vi "Animation Background Thread.vi"(8 "error in (no error)":errorcluster) -> (0 "error out":errorcluster)   [LabVIEW 2017, in "3D Comet.lvclass"]
uses:
  <vilib>/Math Plots/3D Math Plots/3D Comet/3D Comet/3D Comet.lvclass
  <vilib>/Utility/miscctls.llb/LV3DPointTypeDef.ctl
panel:
  in  "Color Array":cluster{"R":sgl, "G":sgl, "B":sgl, "A":sgl}[](array[cluster])
  in  "Body Object":refnum<vi>
  in  "Vertex Array":cluster{"X":sgl, "Y":sgl, "Z":sgl}[](array[cluster])
  in  "3D Scene Ref":refnum<vi>
  in  "Head Object":refnum<vi>
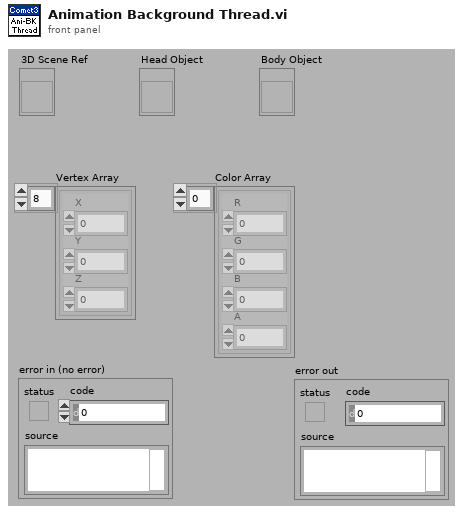
[diagram p1: front panel]
types:
  T1 = typedef "LV3DPointTypeDef.ctl" = cluster{"X":sgl, "Y":sgl, "Z":sgl}
  T2 = enum16{"Overall", "Per Primitive", "Per Vertex", "Binding Off"}
  T3 = enum16{"Points", "Lines", "Line Strip", "Line Loop", "Triangles", "Triangle Strip", "Triangle Fan", "Quads", "Quad Strip", "Polygon"}
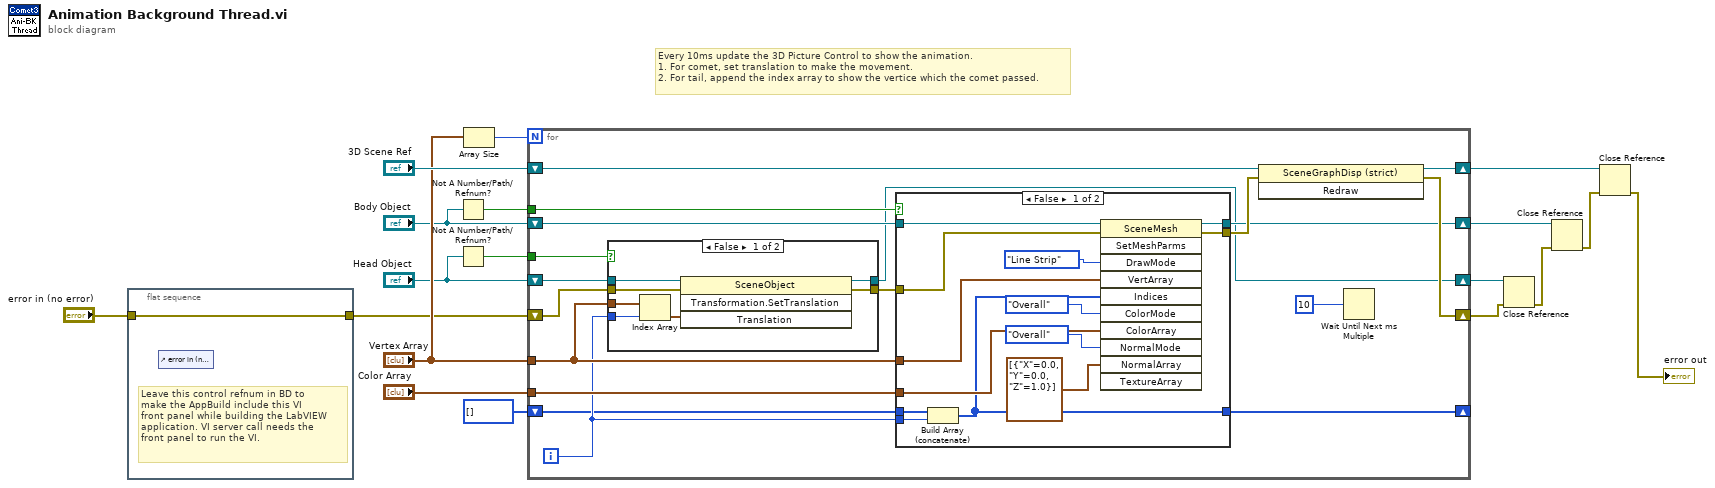
[diagram p0: block diagram]
diagram:
  # "Every 10ms update the 3D Picture Control to show the animation.\n1. For comet, set translation to make the movement.\n2. For tail, append the index array to show the vertice which the comet passed."
  n1 = flat-sequence {
    tunnel: [w19] -> w2
    tunnel: "error in (no error)" -> [w19]
    frame #0 {
      # "Leave this control refnum in BD to \nmake the AppBuild include this VI\nfront panel while building the LabVIEW\napplication. VI server call needs the \nfront panel to run the VI."
      n2 = control-ref of="error in (no error)"() -> ()  [unwired: 1 out]
    }
  }
  n3 = Not A Number/Path/Refnum?(number/path/refnum="Body Object") -> (NaN/Path/Refnum?=w10:bool)
  n4 = Not A Number/Path/Refnum?(number/path/refnum="Head Object") -> (NaN/Path/Refnum?=w11:bool)
  n5 = Array Size(array="Vertex Array") -> (size(s)=w15:i32)
  n6 = for {
    N: w15 -> [_]
    tunnel: "Vertex Array" -> [w33]
    tunnel: "Color Array" -> [w32]
    shift-right: [w25] -> w6
    shift-left: w2 -> [w31]
    shift-right: [w28] -> _
    shift-left: i32[] [] -> [w29]
    tunnel: w11 -> [w24]
    tunnel: w10 -> [w23]
    shift-right: [w22] -> w8
    shift-left: "Body Object" -> [w34]
    shift-right: [w21] -> w9
    shift-left: "3D Scene Ref" -> [w27]
    shift-right: [w20] -> w7
    shift-left: "Head Object" -> [w37]
    i -> [w30]
    n7 = case shown="False" w24 {
      tunnel: w37 -> [w60 w61]
      tunnel: [w59 w62] -> w35
      tunnel: w33 -> [w58 _]
      tunnel: w31 -> [w57 w62]
      tunnel: w30 -> [w55 _]
      tunnel: [w54 w61] -> w20
      frame False {
        n8 = Index Array(array=w58, index=w55) -> (element=w56:cluster{"X":sgl, "Y":sgl, "Z":sgl})
        n9 = invoke class="SceneObject" method="Transformation.SetTranslation"(reference=w60, error in=w57, "Translation"=w56) -> (reference out=w54:refnum<vi>, error out=w59:errorcluster)  [unwired: 1 in, 2 out]
      }
      frame True {
      }
    }
    n10 = case shown="False" w23 {
      tunnel: w35 -> [w50 w52]
      tunnel: w34 -> [w49 w51]
      tunnel: w33 -> [w47 _]
      tunnel: w32 -> [w46 _]
      tunnel: w30 -> [w44 _]
      tunnel: w29 -> [w43 w53]
      tunnel: [w42 w53] -> w28
      tunnel: [w41 w52] -> w26
      tunnel: [w38 w51] -> w22
      frame False {
        n11 = Build Array (concatenate)(w43, w44) -> (w42:i32[])
        n12 = invoke class="SceneMesh" method="SetMeshParms"(reference=w49, error in=w50, "DrawMode"=T3."Line Strip" ("Draw Mode"), "VertArray"=w47, "Indices"=w42, "ColorMode"=T2."Overall" ("Color Binding Mode"), "ColorArray"=w46, "NormalMode"=T2."Overall" ("Normal Binding Mode"), "NormalArray"=T1[] [{"X"=0.0, "Y"=0.0, "Z"=1.0}] ("Normal Array")) -> (reference out=w38:refnum<vi>, error out=w41:errorcluster)  [unwired: 2 in, 9 out]
      }
      frame True {
      }
    }
    n13 = invoke class="SceneGraphDisp (strict)" method="Redraw"(reference=w27, error in=w26) -> (reference out=w21:refnum<vi>, error out=w25:errorcluster)  [unwired: 1 in, 1 out]
    n14 = Wait Until Next ms Multiple(millisecond multiple=u32 10 ("milliseconds to wait")) -> ()  [unwired: 1 out]
  }
  n15 = Close Reference(reference=w7, error in (no error)=w6) -> (error out=w5:errorcluster)
  n16 = Close Reference(reference=w8, error in (no error)=w5) -> (error out=w4:errorcluster)
  n17 = Close Reference(reference=w9, error in (no error)=w4) -> (error out=→"error out":errorcluster)
